vi "Convert_String_to_TimeStamp_me.vi"(1 "string timestamp":string) -> (0 "seconds":u32)   [LabVIEW 2010]
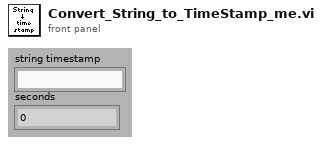
[diagram p1: front panel]
types:
  T1 = cluster{i32, i32, i32, i32, i32, i32, i32, i32, i32}
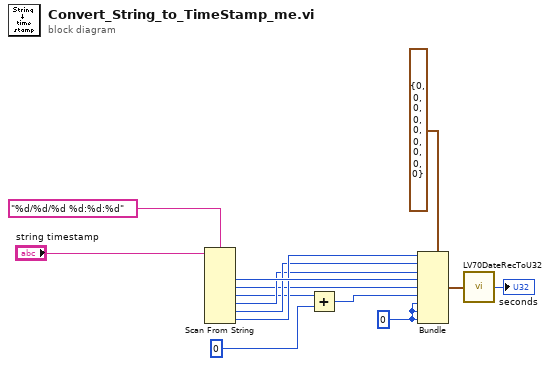
[diagram p0: block diagram]
diagram:
  w7 = 0 ("element")
  n1 = Scan From String(format string="%d/%d/%d %d:%d:%d", input string="string timestamp") -> (output 1=w11:i32, output 2=w4:i32, output 3=w3:i32, output 4=w8:i32, output 5=w9:i32, output 6=w10:i32)  [unwired: 2 in, 9 out]
  n2 = Add(x=w3, y=0) -> (x+y=w1:i32)
  n3 = Bundle(cluster=T1 {0, 0, 0, 0, 0, 0, 0, 0, 0} ("input cluster"), w10, w9, w8, w11, w4, w1, w7, w7, w7) -> (w6:T1)
  n4 = call <vilib>:"LV70DateRecToU32.vi"("date time rec"=w6) -> ("Time"=→"seconds":u32)
